vi "Tosca-Initialize Input Events.vi"(0 "Input Events":T2[](array[typedef]), 7 "Flags":T1[](array[typedef]), 11 "error in (no error)":errorcluster) -> (4 "Input Events Out":T2[](array[typedef]), 15 "error IO":errorcluster)   [LabVIEW 2020]
uses:
  Tosca-Input Event.ctl
  Tosca-Input Criterion.ctl
  epl-vi-lib/Utility VIs/Type Defs/Logic State.ctl
  Typedefs/Tosca-Accumulator.ctl
  Typedefs/Tosca-Flag.ctl
  Sub VIs/Tosca-Globals.vi
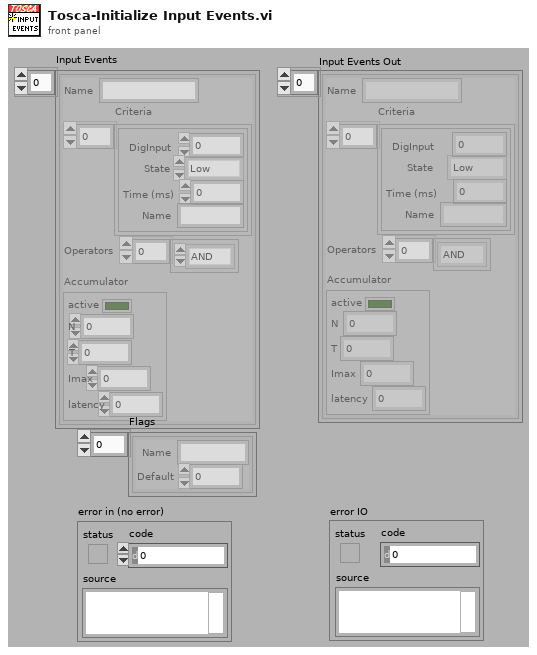
[diagram p1: front panel]
types:
  T1 = typedef "Tosca-Flag.ctl" = cluster{"Name":string, "Default":i32}
  T2 = typedef "Tosca-Input Event.ctl" = cluster{"Name":string, "Criteria":T3[], "Operators":enum16{"AND", "OR"}[], "Accumulator":T5}
  T3 = typedef "Tosca-Input Criterion.ctl" = cluster{"DigInput":i32, "State":T4, "Time (ms)":i32, "Name":string}
  T4 = typedef "Logic State.ctl" = enum16{"Low", "High", "Rising", "Falling"}
  T5 = typedef "Tosca-Accumulator.ctl" = cluster{"active":bool, "N":i32, "T":dbl, "Imax":dbl, "latency":dbl}
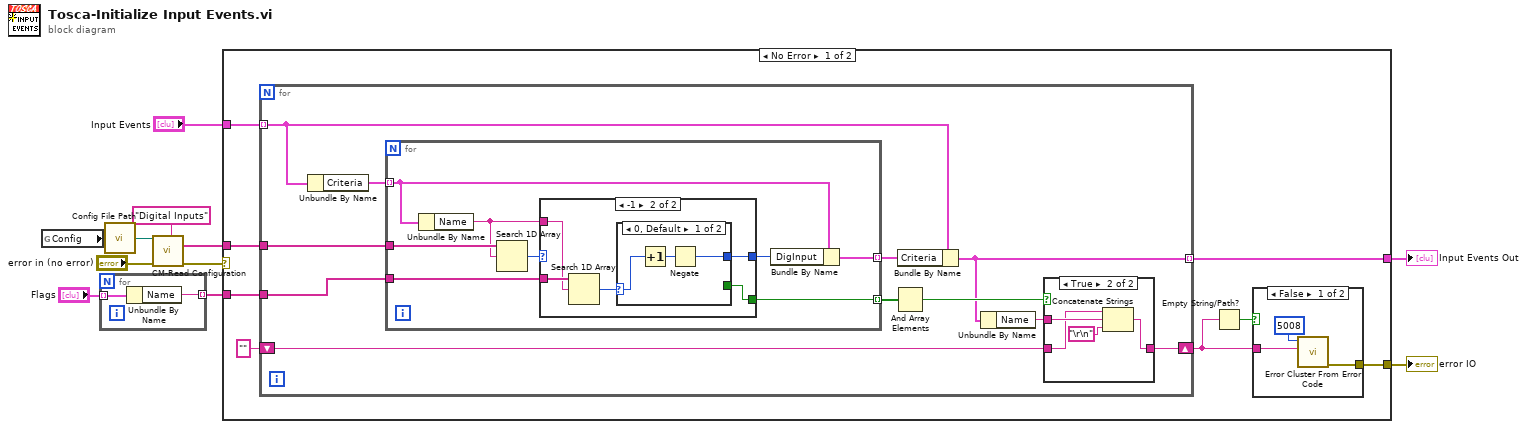
[diagram p0: block diagram]
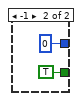
[diagram p3: hidden frame]
diagram:
  n1 = global read "Tosca-Globals.vi" "Config"() -> (w6:string)
  n2 = for {
    tunnel: "Flags" -> [w13] mode=indexing
    tunnel: [w12] -> w7 mode=indexing
    n3 = Unbundle By Name(w13) -> ("Name"=w12:string)
  }
  n4 = call "Config File Path.vi"("AppName"=w6) -> ("Default config file name"=w4:path)
  n5 = call "CM-Read Configuration.vi"("Connection File Path"=w4, "Section"="Digital Inputs", "error in (no error)"="error in (no error)") -> ("Names"=w3:string[], "error out"=w1:errorcluster)  [unwired: 8 in, 3 out]
  n6 = case shown="No Error" w1 {
    selector: w1 -> [_ w61]
    tunnel: w3 -> [w20 _]
    tunnel: "Input Events" -> [w21 w60]
    tunnel: [w15 w61] -> w10
    tunnel: [w18 w60] -> w9
    tunnel: w7 -> [w14 _]
    frame No Error {
      n7 = for {
        tunnel: w21 -> [w31] mode=indexing
        tunnel: w20 -> [w32]
        tunnel: [w28] -> w18 mode=indexing
        shift-right: [w26] -> w16
        shift-left: "" -> [w25]
        tunnel: w14 -> [w22]
        n8 = Unbundle By Name(w31) -> ("Criteria"=w24:T3[])
        n9 = for {
          tunnel: w24 -> [w39] mode=indexing
          tunnel: w32 -> [w40]
          tunnel: [w38] -> w23 mode=indexing
          tunnel: [w35] -> w30 mode=indexing
          tunnel: w22 -> [w34]
          n10 = Unbundle By Name(w39) -> ("Name"=w33:string)
          n11 = Search 1D Array(1D array=w40, element=w33) -> (index of element=w37:i32)  [unwired: 1 in]
          n12 = case shown="-1" w37 {
            selector: w37 -> [w41 _]
            tunnel: [w41 w42] -> w36
            tunnel: [_ w43] -> w35
            tunnel: w34 -> [_ w46]
            tunnel: w33 -> [_ w45]
            frame 0, Default {
            }
            frame -1 {
              n13 = Search 1D Array(1D array=w46, element=w45) -> (index of element=w44:i32)  [unwired: 1 in]
              n14 = case shown="0, Default" w44 {
                selector: w44 -> [w49 _]
                tunnel: [_ TRUE] -> w43
                tunnel: [w47 0] -> w42
                frame 0, Default {
                  n15 = Increment(x=w49) -> (x+1=w48:i32)
                  n16 = Negate(x=w48) -> (-x=w47:i32)
                }
                frame -1 {
                }
              }
            }
          }
          n17 = Bundle By Name(cluster=w39, "DigInput"=w36) -> (w38:T3)
        }
        n18 = And Array Elements(Boolean array=w30) -> (logical AND=w29:bool)
        n19 = Bundle By Name(cluster=w31, "Criteria"=w23) -> (w28:T2)
        n20 = Unbundle By Name(w28) -> ("Name"=w27:string)
        n21 = case shown="True" w29 {
          tunnel: w27 -> [_ w56]
          tunnel: [w52 w54] -> w26
          tunnel: w25 -> [w52 w53]
          frame False {
          }
          frame True {
            n22 = Concatenate Strings(w53, w56, "\r\n") -> (w54:string)
          }
        }
      }
      n23 = Empty String/Path?(string/path=w16) -> (empty?=w17:bool)
      n24 = case shown="False" w17 {
        tunnel: w16 -> [w59 _]
        tunnel: [w58 _] -> w15
        frame False {
          n25 = call <vilib>:"Error Cluster From Error Code.vi"("error message (\"\")"=w59, "error code (0)"=5008) -> ("error out"=w58:errorcluster)  [unwired: 7 in]
        }
        frame True {
        }
      }
    }
    frame Error {
    }
  }
  "error IO" <- w10
  "Input Events Out" <- w9
